vi "Write Bookmark to XML.vi"(2 "Type":T1, 5 "PDF path file":path, 7 "XML File":path, 11 "error in (no error)":errorcluster) -> (8 "XML File duplicate":path, 15 "error out":errorcluster)   [LabVIEW 2019]
doc: "Version 1.1\nDeveloped by Jean-Marc Simard\nCopyright © 2012, Exaprom Inc.\nAll rights reserved.\nLicense: BSD\n\nWith iTextSharp 4.1.6 (http://itextsharp.sourceforge.net)\nunder Mozilla Public License Version 1.1\n(http://www.mozilla.org/MPL/MPL-1.1.html)"
uses:
  <userlib>/Exaprom PDF/Controls/Text Controls/Unicode/Character type.ctl
  <userlib>/Exaprom PDF/Controls/General Controls/Create, open or close.ctl
  <userlib>/Exaprom PDF/Controls/Concatenate Controls/PDF file to concatenate.ctl
  C:/Program Files/National Instruments/LabVIEW 2019/user.lib/Exaprom PDF/DLL/itextsharp.dll
  DLL/itextsharp.dll
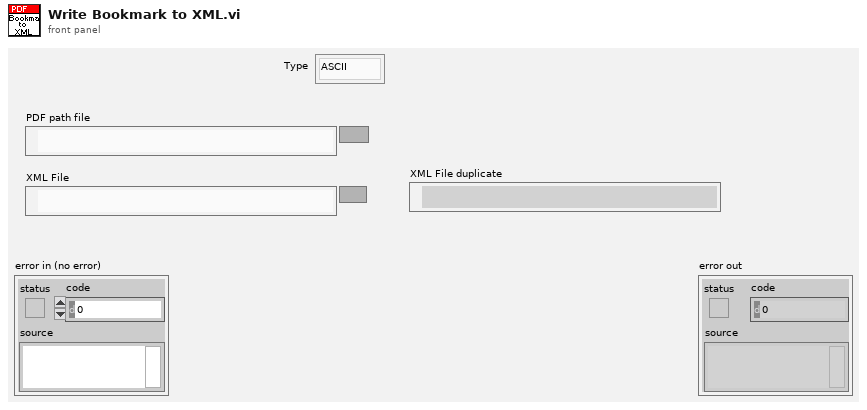
[diagram p1: front panel]
types:
  T1 = typedef "Character type.ctl" = enum16{"ASCII", "Unicode"}
  T2 = typedef "PDF file to concatenate.ctl" = cluster{"Path":path, "Pages":string, "Password":string}
  T3 = typedef "Create, open or close.ctl" = enum16{"Create", "Open", "Close"}
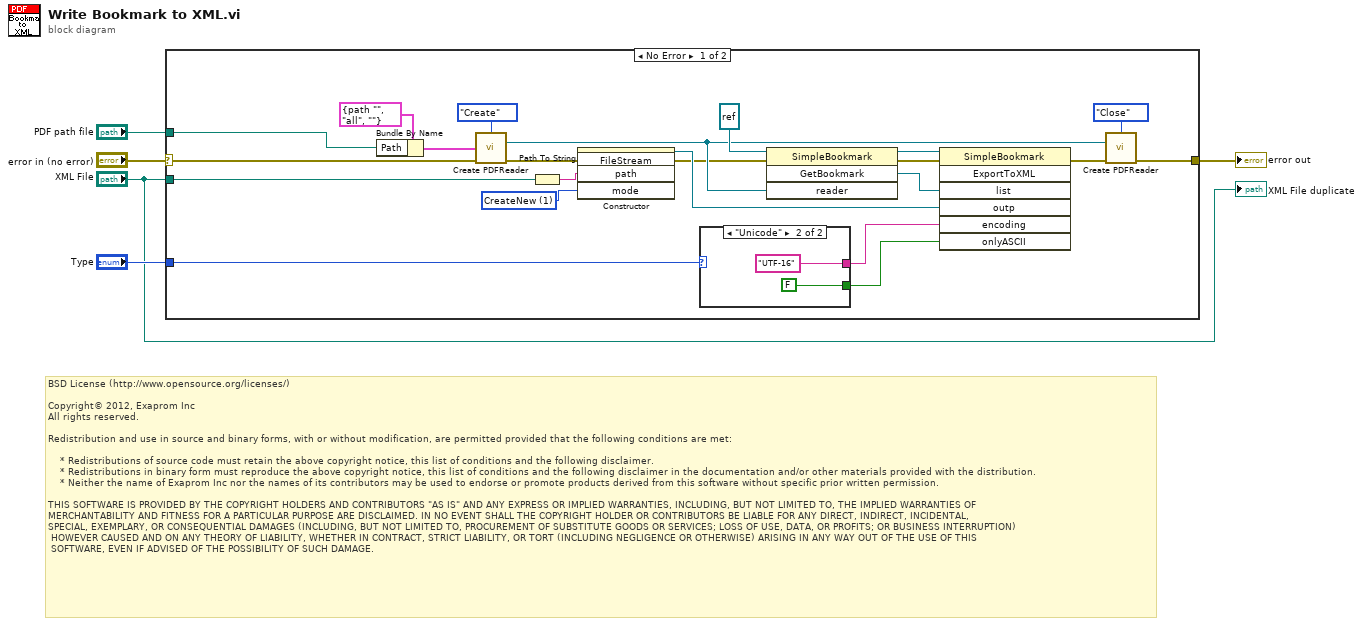
[diagram p0: block diagram]
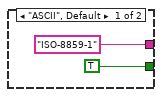
[diagram p2: hidden frame]
diagram:
  # "BSD License (http://www.opensource.org/licenses/)\n\nCopyright© 2012, Exaprom Inc\nAll rights reserved.\n\nRedistribution and use in source and binary forms, with or without modification, are permitted provided that the following conditions are met:\n\n    * Redistributions of source code must retain the above copyright notice, this list of conditions and the following disclaimer.\n    * Redistributions in binary form must reproduce the above copyright notice, this list of conditions and the following disclaimer in the documentation and/or other materials provided with the distribution.\n    * Neither the name of Exaprom Inc nor the names of its contributors may be used to endorse or promote products derived from this software without specific prior written permission.\n\nTHIS SOFTWARE IS PROVIDED BY THE COPYRIGHT HOLDERS AND CONTRIBUTORS \"AS IS\" AND ANY EXPRESS OR IMPLIED WARRANTIES, INCLUDING, BUT NOT LIMITED TO, THE IMPLIED WARRANTIES OF \nMERCHANTABILITY AND FITNESS FOR A PARTICULAR PURPOSE ARE DISCLAIMED. IN NO EVENT SHALL THE COPYRIGHT HOLDER OR CONTRIBUTORS BE LIABLE FOR ANY DIRECT, INDIRECT, INCIDENTAL,\nSPECIAL, EXEMPLARY, OR CONSEQUENTIAL DAMAGES (INCLUDING, BUT NOT LIMITED TO, PROCUREMENT OF SUBSTITUTE GOODS OR SERVICES; LOSS OF USE, DATA, OR PROFITS; OR BUSINESS INTERRUPTION)\n HOWEVER CAUSED AND ON ANY THEORY OF LIABILITY, WHETHER IN CONTRACT, STRICT LIABILITY, OR TORT (INCLUDING NEGLIGENCE OR OTHERWISE) ARISING IN ANY WAY OUT OF THE USE OF THIS\n SOFTWARE, EVEN IF ADVISED OF THE POSSIBILITY OF SUCH DAMAGE."
  n1 = case shown="No Error" "error in (no error)" {
    selector: "error in (no error)" -> [w8 w32]
    tunnel: [w7 w32] -> w5
    tunnel: "PDF path file" -> [w12 _]
    tunnel: "XML File" -> [w9 _]
    tunnel: "Type" -> [w6 _]
    frame No Error {
      w17 = 1 items=["CreateNew"=1, "Create"=2, "Open"=3, "OpenOrCreate"=4, "Truncate"=5, "Append"=6] ("mode")
      n2 = Bundle By Name(cluster=T2 {"Path"=path "", "Pages"="all", "Password"=""} ("File and pages"), "Path"=w12) -> (w13:T2)
      n3 = call <userlib>:"Create PDFReader.vi"("Action"=Create,_open_or_close."Create", "File and pages"=w13, "error in (no error)"=w8) -> ("PdfReader OUT"=w24:refnum<k24>, "error out"=w10:errorcluster)  [unwired: 9 in, 2 out]
      n4 = Path To String(path=w9) -> (string=w18:string)
      n5 = constructor class="FileStream" ("Constructor Node")(error in=w10, "path"=w18, "mode"=w17) -> (reference out=w16:refnum<k24>, error out=w11:errorcluster)  [unwired: 2 in, 3 out]
      n6 = case shown="\"Unicode\"" w6 {
        tunnel: ["ISO-8859-1" ("encoding") "UTF-16" ("encoding")] -> w21
        tunnel: [TRUE ("onlyASCII") FALSE ("onlyASCII")] -> w20
        frame "ASCII", Default {
        }
        frame "Unicode" {
        }
      }
      n7 = invoke class="SimpleBookmark" method="GetBookmark"(reference=refnum<k24> refnum ("new reference"), error in=w11, "reader"=w24) -> (reference out=w23:refnum<k24>, error out=w22:errorcluster, "GetBookmark"=w15:refnum<k24>)  [unwired: 1 in, 1 out]
      n8 = invoke class="SimpleBookmark" method="ExportToXML"(reference=w23, error in=w22, "list"=w15, "outp"=w16, "encoding"=w21, "onlyASCII"=w20) -> (error out=w19:errorcluster)  [unwired: 1 in, 6 out]
      n9 = call <userlib>:"Create PDFReader.vi"("Action"=Create,_open_or_close."Close", "PdfReader IN"=w24, "error in (no error)"=w19) -> ("error out"=w7:errorcluster)  [unwired: 9 in, 3 out]
    }
    frame Error {
    }
  }
  "error out" <- w5
  "XML File duplicate" <- "XML File"
